vi "Sample_Scan_Pause_Para.vi"(8 "Z tilt comp":bool, 9 "Microsteps (MS=64)":dbl=64.0, 10 "Tilt x/z":dbl=64.0, 11 "waypoints path":path=path "C:/Users/ALS Measurement/Google Drive/LabVIEW/Thermionics Manipulator") -> (0 "Delta M2 in plain total":dbl, 1 "Delta M1 in plain total":dbl, 2 "M2 Z tilt comp total":dbl, 3 "Delta M3 total":dbl, 4 "Problem":bool, 5 "tilt angle (rad)":dbl, 6 "Top Left Position Array":i32[](array[numeric]), 7 "in plain angle (rad)":dbl)   [LabVIEW 2018]
uses:
  ConversionAndInformation/Unit_Control.ctl
panel:
  out "x/z":dbl
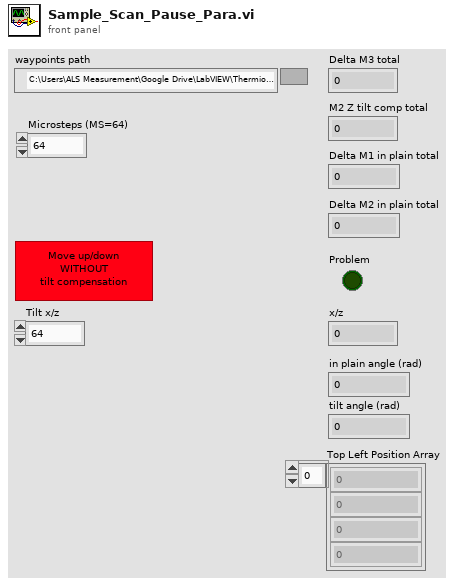
[diagram p1: front panel]
types:
  T1 = typedef "Unit_Control.ctl" = enum16{"Angle (Degrees)", "Rad", "Angle [TMC]", "Microsteps [TMC]", "Inches", "Nanometer", "Meter", "Centimeter", "Millimeter", "Micron"}
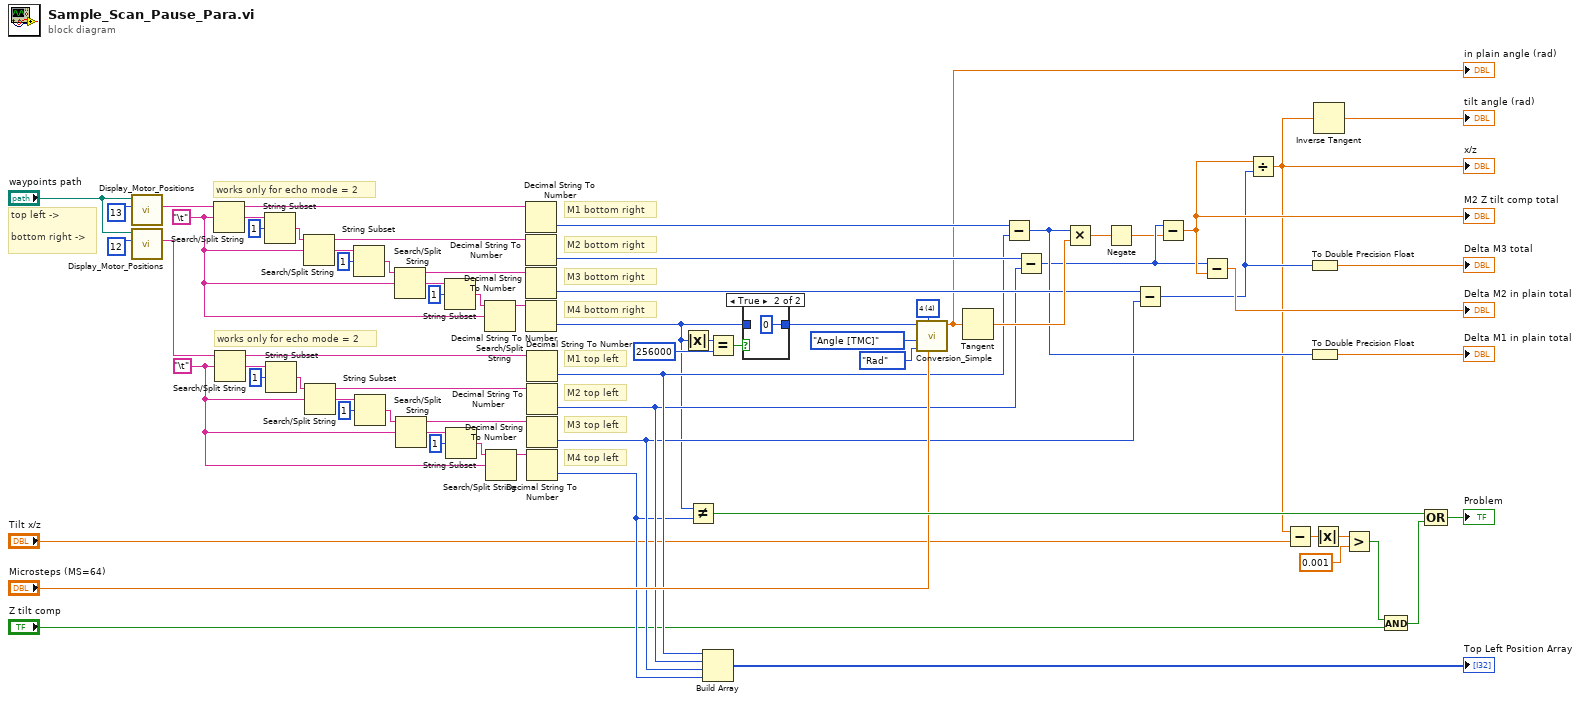
[diagram p0: block diagram]
diagram:
  w35 = u16 4 items=["none", "1", "2", "3", "4", "all"] ("Motor")
  w41 = "\t"
  w69 = "\t"
  # "M3 bottom right"
  # "M4 bottom right"
  # "M2 bottom right"
  # "M1 bottom right"
  # "M4 top left"
  # "M3 top left"
  # "M2 top left"
  # "M1 top left"
  # "works only for echo mode = 2"
  # "works only for echo mode = 2"
  # "top left ->\n\nbottom right ->"
  n1 = call "Display_Motor_Positions.vi"("Waypoint Number"=13, "base path"="waypoints path") -> ("Loaded Positions"=w55:string)  [unwired: 8 in, 1 out]
  n2 = call "Display_Motor_Positions.vi"("Waypoint Number"=12, "base path"="waypoints path") -> ("Loaded Positions"=w40:string)  [unwired: 8 in, 1 out]
  n3 = Search/Split String(string=w55, search string/char (-)=w69) -> (substring before match=w59:string, match + rest of string=w60:string)  [unwired: 1 in, 1 out]
  n4 = Search/Split String(string=w40, search string/char (-)=w41) -> (substring before match=w51:string, match + rest of string=w50:string)  [unwired: 1 in, 1 out]
  n5 = String Subset(string=w60, offset (0)=1) -> (substring=w61:string)  [unwired: 1 in]
  n6 = String Subset(string=w50, offset (0)=1) -> (substring=w49:string)  [unwired: 1 in]
  n7 = Search/Split String(string=w61, search string/char (-)=w69) -> (substring before match=w58:string, match + rest of string=w63:string)  [unwired: 1 in, 1 out]
  n8 = Search/Split String(string=w49, search string/char (-)=w41) -> (substring before match=w52:string, match + rest of string=w47:string)  [unwired: 1 in, 1 out]
  n9 = String Subset(string=w63, offset (0)=1) -> (substring=w64:string)  [unwired: 1 in]
  n10 = String Subset(string=w47, offset (0)=1) -> (substring=w46:string)  [unwired: 1 in]
  n11 = Search/Split String(string=w64, search string/char (-)=w69) -> (substring before match=w57:string, match + rest of string=w67:string)  [unwired: 1 in, 1 out]
  n12 = Search/Split String(string=w46, search string/char (-)=w41) -> (substring before match=w53:string, match + rest of string=w43:string)  [unwired: 1 in, 1 out]
  n13 = String Subset(string=w67, offset (0)=1) -> (substring=w68:string)  [unwired: 1 in]
  n14 = String Subset(string=w43, offset (0)=1) -> (substring=w42:string)  [unwired: 1 in]
  n15 = Search/Split String(string=w68, search string/char (-)=w69) -> (substring before match=w56:string)  [unwired: 1 in, 2 out]
  n16 = Search/Split String(string=w42, search string/char (-)=w41) -> (substring before match=w54:string)  [unwired: 1 in, 2 out]
  n17 = Decimal String To Number(string=w59) -> (number=w33:i32)  [unwired: 2 in, 1 out]
  n18 = Decimal String To Number(string=w58) -> (number=w31:i32)  [unwired: 2 in, 1 out]
  n19 = Decimal String To Number(string=w57) -> (number=w30:i32)  [unwired: 2 in, 1 out]
  n20 = Decimal String To Number(string=w56) -> (number=w5:i32)  [unwired: 2 in, 1 out]
  n21 = Decimal String To Number(string=w51) -> (number=w21:i32)  [unwired: 2 in, 1 out]
  n22 = Decimal String To Number(string=w52) -> (number=w20:i32)  [unwired: 2 in, 1 out]
  n23 = Decimal String To Number(string=w53) -> (number=w19:i32)  [unwired: 2 in, 1 out]
  n24 = Decimal String To Number(string=w54) -> (number=w18:i32)  [unwired: 2 in, 1 out]
  n25 = Absolute Value(x=w5) -> (abs(x)=w8:i32)
  n26 = Not Equal?(x=w5, y=w18) -> (x != y?=w39:bool)
  n27 = Build Array(w21, w20, w19, w18) -> (→"Top Left Position Array":i32[])
  n28 = Equal?(x=w8, y=256000) -> (x = y?=w6:bool)
  n29 = case shown="True" w6 {
    tunnel: w5 -> [w73 _]
    tunnel: [w73 0] -> w4
    frame False {
    }
    frame True {
    }
  }
  n30 = call "Conversion_Simple.vi"("Microsteps (MS=64)"="Microsteps (MS=64)", "Motor"=w35, "Output Unit"=Unit_Control."Rad", "Input Unit"=Unit_Control."Angle [TMC]", "Input"=w4) -> ("Output"=w23:dbl)  [unwired: 5 in, 1 out]
  "in plain angle (rad)" <- w23
  n31 = Tangent(1:w23) -> (0:w32:dbl)
  n32 = Subtract(x=w33, y=w21) -> (x-y=w27:i32)
  n33 = Subtract(x=w31, y=w20) -> (x-y=w16:i32)
  n34 = Multiply(x=w27, y=w32) -> (x*y=w15:dbl)
  n35 = Negate(x=w15) -> (-x=w14:dbl)
  n36 = Subtract(x=w30, y=w19) -> (x-y=w25:i32)
  n37 = Subtract(x=w16, y=w14) -> (x-y=w29:dbl)
  "M2 Z tilt comp total" <- w29
  n38 = Subtract(x=w16, y=w29) -> (x-y=→"Delta M2 in plain total":dbl)
  n39 = Divide(x=w29, y=w25) -> (x/y=w13:dbl)
  "x/z" <- w13
  n40 = Subtract(x=w13, y="Tilt x/z") -> (x-y=w11:dbl)
  n41 = To Double Precision Float(number=w25) -> (double precision float=→"Delta M3 total":dbl)
  n42 = To Double Precision Float(number=w27) -> (double precision float=→"Delta M1 in plain total":dbl)
  n43 = Absolute Value(x=w11) -> (abs(x)=w10:dbl)
  n44 = Inverse Tangent(1:w13) -> (0:→"tilt angle (rad)":dbl)
  n45 = Greater?(x=w10, y=0.001) -> (0:w3:bool)
  n46 = And(x=w3, y="Z tilt comp") -> (x .and. y?=w1:bool)
  n47 = Compound Arithmetic op=OR(w39, w1) -> (→"Problem":bool)
